vi "ConvertI16FXP.vi"(1 "I16":i16) -> (0 "y":fxp<+/-,16,16>)   [LabVIEW 2025]
uses:
  <vilib>/rvi/FXPMathLib/FxpInterpret/XNode/nifxpmath_Interpret.xnode
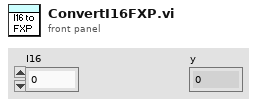
[diagram p1: front panel]
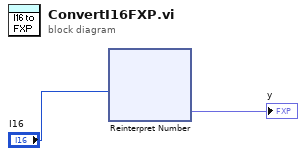
[diagram p0: block diagram]
diagram:
  n1 = xnode "Reinterpret Number"("x"="I16") -> ("y"=→"y":fxp<+/-,16,16>)
